vi "conv_Float_To_Word.vi"(11 "input_Float":sgl) -> (0 "second_Word":u16, 3 "first_Word":u16)   [LabVIEW 2023, in "pump_Lib.lvlib"]
uses:
  pump_Lib.lvlib
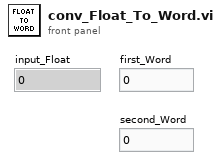
[diagram p1: front panel]
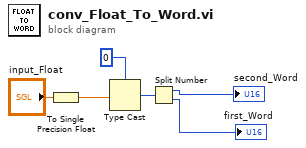
[diagram p0: block diagram]
diagram:
  n1 = To Single Precision Float(number="input_Float") -> (single precision float=w4:sgl)
  n2 = Type Cast(type=u32 0 ("(hi.lo)"), x=w4) -> (*(type *) &x=w3:u32)
  n3 = Split Number(x=w3) -> (hi(x)=→"second_Word":u16, lo(x)=→"first_Word":u16)
